vi "Timescale_Factor.vi"() -> (0 "Factor to scale timescale by":dbl)   [LabVIEW 2010]
panel:
  # "See Diagram for Value"
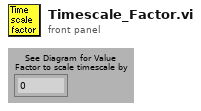
[diagram p1: front panel]
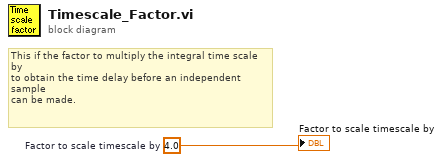
[diagram p0: block diagram]
diagram:
  w1 = 4.0  # Factor to scale timescale by
  # "This if the factor to multiply the integral time scale by\nto obtain the time delay before an independent sample\ncan be made."
  "Factor to scale timescale by" <- w1
